vi "Config-Stress-Channel.vi"(0 "VISA session":refnum<visa-resource-name>, 1 "PGU mode\n(V:0)":u16(ring) items=["V", "V pulse"], 2 "compliance\n(SMU only)":dbl=0.1 format="%^.2e", 5 "unit (VSU1:0)":u16(ring) items=["VSU1", "VSU2", "SMU1", "SMU2", "SMU3", "SMU4", "SMU5", "SMU6", "PGU1", "PGU2", "GNDU"], 7 "source\n(SMU/PGU/VSU)":dbl=0.01 format="%^.2e", 9 "function (com:0)":u16(ring) items=["disable", "sync", "nsync"], 11 "error in (no error)":errorcluster, 12 "SMU mode\n(common:0)":u16(ring) items=["common", "V", "I"], 13 "name (max 6 chars)":string) -> (4 "VISA resource name out":refnum<visa-resource-name>, 15 "error out":errorcluster)   [LabVIEW 2016, in "Agilent 415X Series.lvlib"]
doc: "This VI configures a unit for stress operation. Allowed units are\nPGU1-2, GNDU, SMU1-6 and VSU 1-2."
uses:
  Agilent 415X Series.lvlib
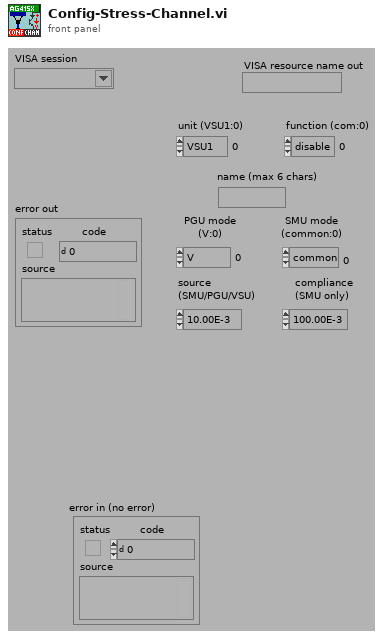
[diagram p1: front panel]
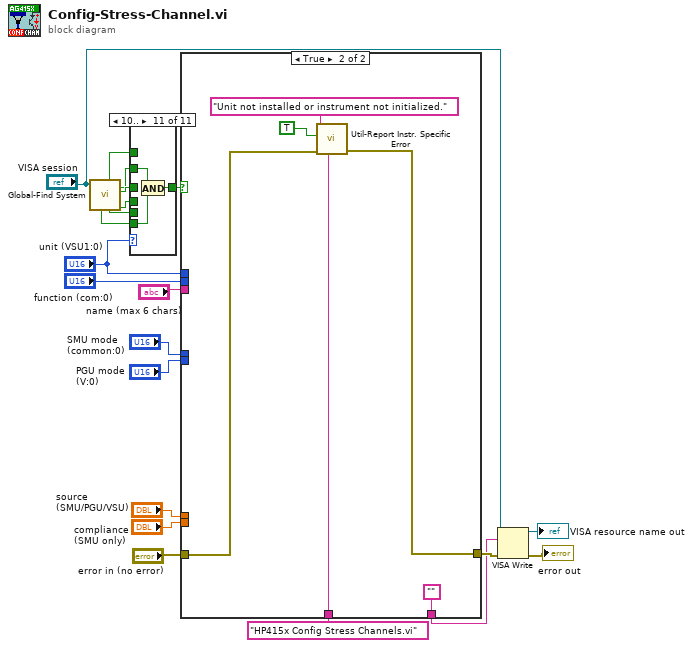
[diagram p0: block diagram]
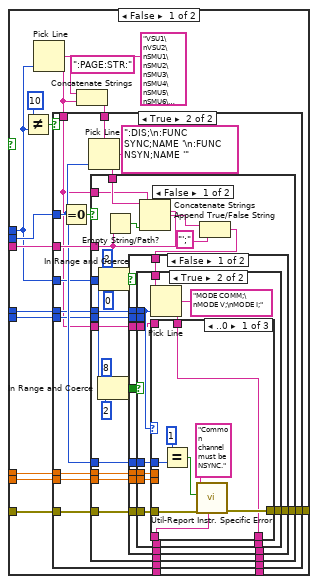
[diagram p2: hidden frame]
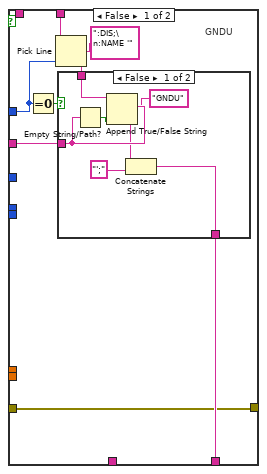
[diagram p3: hidden frame]
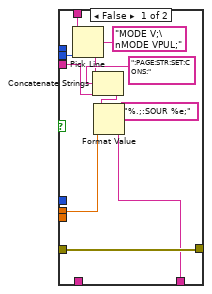
[diagram p5: hidden frame]
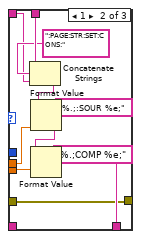
[diagram p6: hidden frame]
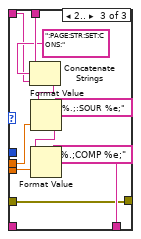
[diagram p7: hidden frame]
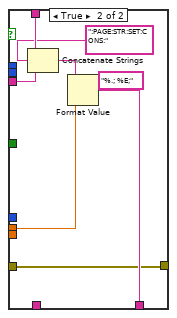
[diagram p8: hidden frame]
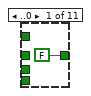
[diagram p10: hidden frame]
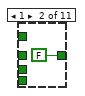
[diagram p11: hidden frame]
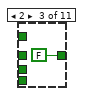
[diagram p12: hidden frame]
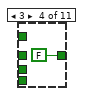
[diagram p13: hidden frame]
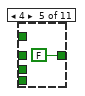
[diagram p14: hidden frame]
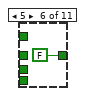
[diagram p15: hidden frame]
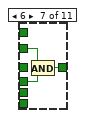
[diagram p16: hidden frame]
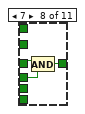
[diagram p17: hidden frame]
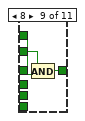
[diagram p18: hidden frame]
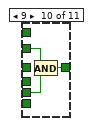
[diagram p19: hidden frame]
diagram:
  n1 = call "Global-Find System.vi"("VISA session"="VISA session") -> ("found"=w17:bool, "SMU6 present"=w15:bool, "PGU2 present"=w18:bool, "PGU1 present"=w16:bool, "GNDU present"=w19:bool, "SMU5 present"=w14:bool)  [unwired: 3 in, 2 out]
  n2 = case shown="10.." "unit (VSU1:0)" {
    tunnel: [FALSE FALSE FALSE FALSE FALSE FALSE w30 w33 w36 w39 w42] -> w13
    tunnel: w14 -> [_ _ _ _ _ _ w29 _ w35 w38 w41]
    tunnel: w15 -> [_ _ _ _ _ _ _ w31 _ _ _]
    tunnel: w16 -> [_ _ _ _ _ _ _ _ w34 _ _]
    tunnel: w17 -> [_ _ _ _ _ _ w28 w32 _ _ _]
    tunnel: w18 -> [_ _ _ _ _ _ _ _ _ w37 _]
    tunnel: w19 -> [_ _ _ _ _ _ _ _ _ _ w40]
    frame ..0 {
    }
    frame 1 {
    }
    frame 2 {
    }
    frame 3 {
    }
    frame 4 {
    }
    frame 5 {
    }
    frame 6 {
      n3 = And(x=w29, y=w28) -> (x .and. y?=w30:bool)
    }
    frame 7 {
      n4 = And(x=w31, y=w32) -> (x .and. y?=w33:bool)
    }
    frame 8 {
      n5 = And(x=w35, y=w34) -> (x .and. y?=w36:bool)
    }
    frame 9 {
      n6 = And(x=w38, y=w37) -> (x .and. y?=w39:bool)
    }
    frame 10.. {
      n7 = And(x=w41, y=w40) -> (x .and. y?=w42:bool)
    }
  }
  n8 = case shown="True" w13 {
    tunnel: "HP415x Config Stress Channels.vi" -> [w45 w196]
    tunnel: "function (com:0)" -> [w56 _]
    tunnel: "name (max 6 chars)" -> [w54 _]
    tunnel: "SMU mode\n(common:0)" -> [w49 _]
    tunnel: "PGU mode\n(V:0)" -> [w48 _]
    tunnel: "unit (VSU1:0)" -> [w50 _]
    tunnel: [w52 "" ("Empty String Constant")] -> w11
    tunnel: "source\n(SMU/PGU/VSU)" -> [w47 _]
    tunnel: "compliance\n(SMU only)" -> [w46 _]
    tunnel: "error in (no error)" -> [w44 w192]
    tunnel: [w43 w191] -> w12
    frame False {
      n9 = Not Equal?(x=10, y=w50) -> (x != y?=w58:bool)
      n10 = Pick Line(multi-line string="VSU1\nVSU2\nSMU1\nSMU2\nSMU3\nSMU4\nSMU5\nSMU6\nPGU1\nPGU2\nGNDU", line index=w50) -> (output string=w51:string)  [unwired: 1 in]
      n11 = Concatenate Strings(":PAGE:STR:", w51) -> (w57:string)
      n12 = case shown="True" w58 {
        tunnel: w57 -> [w67 w91]
        tunnel: w56 -> [w65 w86]
        tunnel: w54 -> [w62 w87]
        tunnel: [w61 w79] -> w52
        tunnel: w51 -> [_ w82]
        tunnel: w50 -> [_ w85]
        tunnel: w49 -> [_ w84]
        tunnel: w48 -> [_ w83]
        tunnel: w47 -> [_ w81]
        tunnel: w46 -> [_ w80]
        tunnel: w45 -> [_ w78]
        tunnel: w44 -> [w60 w77]
        tunnel: [w60 w76] -> w43
        frame False {
          # "GNDU"
          n13 = Equal To 0?(x=w65) -> (x = 0?=w64:bool)
          n14 = Pick Line(string ("")=w67, multi-line string=":DIS;\n:NAME '", line index=w65) -> (output string=w63:string)
          n15 = case shown="False" w64 {
            tunnel: w63 -> [w74 w75]
            tunnel: w62 -> [w72 _]
            tunnel: [w68 w75] -> w61
            frame False {
              n16 = Empty String/Path?(string/path=w72) -> (empty?=w73:bool)
              n17 = Append True/False String(1:w73, 2:w72, 3:"GNDU", 4:w74) -> (0:w70:string)
              n18 = Concatenate Strings(w70, "';") -> (w68:string)
            }
            frame True {
              # "GNDU Function = Disable"
            }
          }
        }
        frame True {
          n19 = Equal To 0?(x=w86) -> (x = 0?=w89:bool)
          n20 = Pick Line(string ("")=w91, multi-line string=":DIS;\n:FUNC SYNC;NAME '\n:FUNC NSYN;NAME '", line index=w86) -> (output string=w88:string)
          n21 = case shown="False" w89 {
            tunnel: w88 -> [w112 w190]
            tunnel: w82 -> [w111 _]
            tunnel: w87 -> [w110 _]
            tunnel: [w98 w190] -> w79
            tunnel: w85 -> [w100 _]
            tunnel: w84 -> [w108 _]
            tunnel: w83 -> [w107 _]
            tunnel: w82 -> [w101 _]
            tunnel: w81 -> [w99 _]
            tunnel: w80 -> [w96 _]
            tunnel: w86 -> [w95 _]
            tunnel: w78 -> [w94 _]
            tunnel: w77 -> [w93 w189]
            tunnel: [w92 w189] -> w76
            frame False {
              n22 = In Range and Coerce(upper limit=8, x=w100, lower limit=2) -> (In Range?=w97:bool)  [unwired: 1 out]
              n23 = In Range and Coerce(upper limit=2, x=w100, lower limit=0) -> (In Range?=w106:bool)  [unwired: 1 out]
              n24 = Empty String/Path?(string/path=w110) -> (empty?=w115:bool)
              n25 = Append True/False String(1:w115, 2:w110, 3:w111, 4:w112) -> (0:w114:string)
              n26 = Concatenate Strings(w114, "';") -> (w109:string)
              n27 = case shown="False" w106 {
                tunnel: w109 -> [w126 w188]
                tunnel: w108 -> [w124 _]
                tunnel: w107 -> [w116 _]
                tunnel: w101 -> [w125 w186]
                tunnel: w99 -> [w123 w185]
                tunnel: [w121 w182] -> w98
                tunnel: w97 -> [w127 _]
                tunnel: w96 -> [w122 _]
                tunnel: w95 -> [w120 _]
                tunnel: w94 -> [w119 _]
                tunnel: w93 -> [w118 w181]
                tunnel: [w117 w181] -> w92
                frame False {
                  n28 = case shown="True" w127 {
                    tunnel: w126 -> [w138 w150]
                    tunnel: w125 -> [w133 w140]
                    tunnel: w124 -> [_ w141]
                    tunnel: w123 -> [w132 w139]
                    tunnel: w122 -> [_ w148]
                    tunnel: [w128 w147] -> w121
                    tunnel: w120 -> [_ w146]
                    tunnel: w119 -> [_ w145]
                    tunnel: w118 -> [w130 w144]
                    tunnel: [w130 w143] -> w117
                    tunnel: w116 -> [w129 _]
                    frame False {
                      n29 = Pick Line(string ("")=w138, multi-line string="MODE V;\nMODE VPUL;", line index=w129) -> (output string=w134:string)
                      n30 = Concatenate Strings(w134, ":PAGE:STR:SET:CONS:", w133) -> (w131:string)
                      n31 = Format Value(string ("")=w131, format string="%.;:SOUR %e;", value (0)=w132) -> (output string=w128:string)
                    }
                    frame True {
                      n32 = Pick Line(string ("")=w150, multi-line string="MODE COMM;\nMODE V;\nMODE I;", line index=w141) -> (output string=w142:string)
                      n33 = case shown="..0" w141 {
                        tunnel: w148 -> [_ w161 w172]
                        tunnel: [w151 w169 w180] -> w147
                        tunnel: w146 -> [w158 _ _]
                        tunnel: w144 -> [w155 w167 w178]
                        tunnel: [w154 w167 w178] -> w143
                        tunnel: w142 -> [w151 w164 w175]
                        tunnel: w140 -> [_ w160 w171]
                        tunnel: w145 -> [w152 _ _]
                        tunnel: w139 -> [_ w159 w170]
                        frame ..0 {
                          n34 = Equal?(x=1, y=w158) -> (x = y?=w156:bool)
                          n35 = call "Util-Report Instr. Specific Error.vi"("source"=w152, "error in (no error)"=w155, "error message"="Common channel must be NSYNC.", "new error"=w156) -> ("error out"=w154:errorcluster)  [unwired: 6 in, 1 out]
                        }
                        frame 1 {
                          n36 = Concatenate Strings(w164, ":PAGE:STR:SET:CONS:", w160) -> (w165:string)
                          n37 = Format Value(string ("")=w165, format string="%.;:SOUR %e;", value (0)=w159) -> (output string=w162:string)
                          n38 = Format Value(string ("")=w162, format string="%.;COMP %e;", value (0)=w161) -> (output string=w169:string)
                        }
                        frame 2.. {
                          n39 = Concatenate Strings(w175, ":PAGE:STR:SET:CONS:", w171) -> (w176:string)
                          n40 = Format Value(string ("")=w176, format string="%.;:SOUR %e;", value (0)=w170) -> (output string=w173:string)
                          n41 = Format Value(string ("")=w173, format string="%.;COMP %e;", value (0)=w172) -> (output string=w180:string)
                        }
                      }
                    }
                  }
                }
                frame True {
                  n42 = Concatenate Strings(w188, ":PAGE:STR:SET:CONS:", w186) -> (w184:string)
                  n43 = Format Value(string ("")=w184, format string="%.; %E;", value (0)=w185) -> (output string=w182:string)
                }
              }
            }
            frame True {
              # "Disabled"
            }
          }
        }
      }
    }
    frame True {
      n44 = call "Util-Report Instr. Specific Error.vi"("source"=w196, "error in (no error)"=w192, "error message"="Unit not installed or instrument not initialized.", "new error"=TRUE) -> ("error out"=w191:errorcluster)  [unwired: 6 in, 1 out]
    }
  }
  n45 = VISA Write(VISA resource name="VISA session", write buffer=w11, error in (no error)=w12) -> (VISA resource name out=→"VISA resource name out":refnum<visa-resource-name>, error out=→"error out":errorcluster)  [unwired: 1 out]
